vi "SendStatus.vi"(8 "error in (no error)":errorcluster {"code" format="Error %.0f"}, 9 "ErrMessage":string, 10 "NoErrMessage":string, 11 "Message Queue":refnum<queue>) -> (0 "error out":errorcluster {"code" format="Error %.0f"}, 2 "MessageOut":string, 3 "dup Message Queue":refnum<queue>)   [LabVIEW 2017]
doc: "This VI is used to send respective error/no error status messages after completion of any code execution desired. Automatic error handling is disabled for this VI to allow the error case statement to exceute and propagate an error message up the calll chain."
uses:
  Configuration/Message Queues/Message Cluster.ctl
  Configuration/globalConstants.vi
  Configuration/Message Queues/Message Queue.lvlib
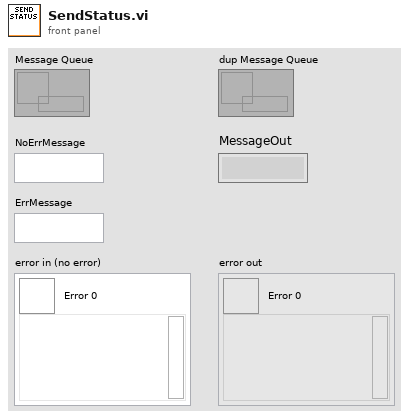
[diagram p1: front panel]
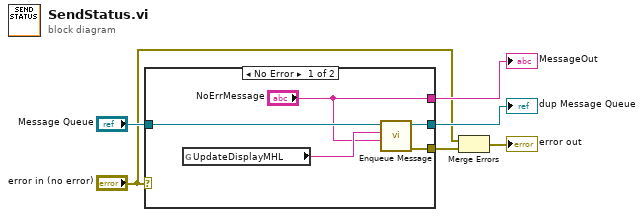
[diagram p0: block diagram]
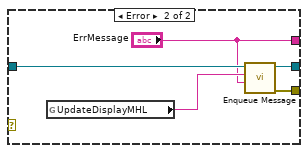
[diagram p2: hidden frame]
diagram:
  n1 = case shown="No Error" "error in (no error)" {
    tunnel: [w11 w16] -> w3
    tunnel: [w10 w15] -> w6
    tunnel: "Message Queue" -> [w9 w14]
    tunnel: ["NoErrMessage" "ErrMessage"] -> w4
    frame No Error {
      n2 = global read "globalConstants.vi" "UpdateDisplayMHL"() -> (w8:string)
      n3 = call "Enqueue Message.vi"("Message Data"="NoErrMessage", "Message"=w8, "Message Queue"=w9) -> ("error out"=w11:errorcluster, "dup Message Queue"=w10:refnum<queue>)  [unwired: 7 in]
    }
    frame Error {
      n4 = global read "globalConstants.vi" "UpdateDisplayMHL"() -> (w13:string)
      n5 = call "Enqueue Message.vi"("Message Data"="ErrMessage", "Message"=w13, "Message Queue"=w14) -> ("error out"=w16:errorcluster, "dup Message Queue"=w15:refnum<queue>)  [unwired: 7 in]
    }
  }
  "dup Message Queue" <- w6
  "MessageOut" <- w4
  n6 = Merge Errors("error in (no error)", w3) -> (→"error out":errorcluster)
